vi "edittest test step configuration.vi"(6 "Write? (f)":bool, 7 "sxTestId (\"\")":string, 8 "error in (no error)":errorcluster, 9 "bConfiguration (to Read for Template Keys) (\"\")":string, 10 "POSTed Step Config (to Write to bConfiguration)\nOR\nTemplate Keys (empty)":T1, 11 "Connection Refnum":T2) -> (0 "error out":errorcluster, 1 "bConfiguration":string, 2 "Template Keys":T1, 3 "Connection Refnum":T2)   [LabVIEW 2011]
uses:
  Summitek EXT/ODBC/SQL Controls/Connection Refnum.ctl
  ITK EXT/utils/keyedarr.llb/Keyed Array.ctl
  tests/Test Function.ctl
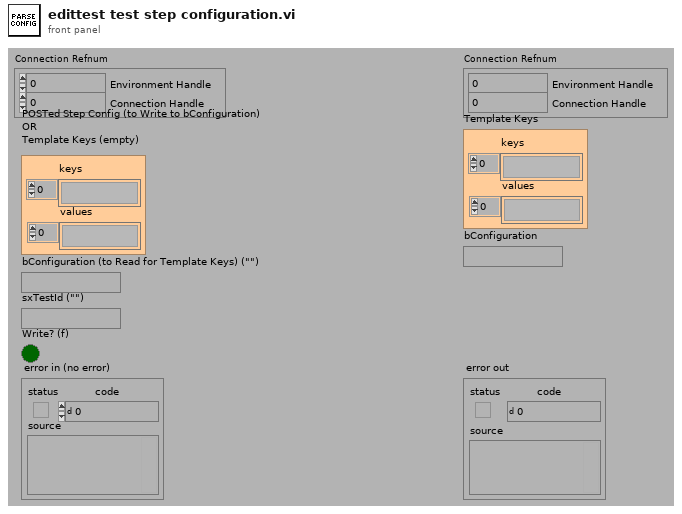
[diagram p1: front panel]
types:
  T1 = typedef "Keyed Array.ctl" = cluster{"keys":string[], "values":string[]}
  T2 = typedef "Connection Refnum.ctl" = cluster{"Environment Handle":i32, "Connection Handle":i32}
  T3 = typedef "Test Function.ctl" = enum16{"Test Config", "Test Storage", "Test Pre-Process", "Unflatten Test Parameters", "Flatten Test Parameters"}
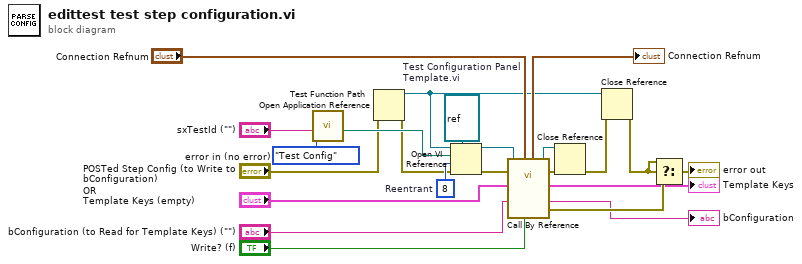
[diagram p0: block diagram]
diagram:
  w22 = 8  # Reentrant
  w18 = refnum<vi> refnum  # Test Configuration Panel Template.vi
  n1 = call "Test Function Path.vi"("Object Type (Test Config)"=Test_Function."Test Config", "Object Name (\"\")"="sxTestId (\"\")") -> ("Object Path"=w19:path)  [unwired: 1 in, 8 out]
  n2 = Open Application Reference(8:"error in (no error)") -> (0:w2:errorcluster, 3:w1:refnum<vi>)  [unwired: 3 in]
  n3 = Open VI Reference(type specifier VI Refnum (for type only)=w18, application reference (local)=w1, vi path=w19, options=w22, error in (no error)=w2) -> (vi reference=w17:refnum<vi>, error out=w13:errorcluster)  [unwired: 1 out]
  n4 = call-by-ref "?"(reference=w17, error in=w13, "Write? (f)"="Write? (f)", "Connection Refnum"="Connection Refnum", "Configuration (\"\")"="bConfiguration (to Read for Template Keys) (\"\")", "Template Keys (empty)"="POSTed Step Config (to Write to bConfiguration)\nOR\nTemplate Keys (empty)") -> (reference out=w16:refnum<vi>, error out=w12:errorcluster, 0:"error out"=w9:errorcluster, "Configuration"=→"bConfiguration":string, "Template Keys"=→"Template Keys":T1, "Connection Refnum"=→"Connection Refnum":T2)  [unwired: 4 in]
  n5 = Close Reference(reference=w16, error in (no error)=w12) -> (error out=w5:errorcluster)
  n6 = Close Reference(reference=w1, error in (no error)=w5) -> (error out=w4:errorcluster)
  n7 = Select(t=w4, s=w4, f=w9) -> (s? t:f=→"error out":errorcluster)
